vi "Write Single Coil1.vi"(7 "Unit_ID":T1, 8 "error in (no error)":errorcluster, 9 "coil value":bool, 10 "address":u16, 11 "Modbus master in":refnum<class "TCP.lvclass">) -> (0 "error out":errorcluster, 3 "Modbus master out":refnum<class "TCP.lvclass">)   [LabVIEW 2019, in "NI_modbus_upd.lvlib"]
doc: "Writes a value to a single coil."
uses:
  NI_modbus_upd.lvlib
  TCP/TCP.lvclass
  Ctl/Unit_ID.ctl
  TCP/TCP.lvclass/TCP.ctl
  Error Generator1.vi
  Function code mismatch error1.vi
  Read ADU Packet Master.vi
  Write ADU Packet Master.vi
  Modbus Data Unit (PDU)/Construct PDU1.vi
  Modbus Data Unit (PDU)/Unflatten to PDU1.vi
  TCP/Protocol Read.vi
  TCP/Protocol Write.vi
  <vilib>/Utility/error.llb/Error Cluster From Error Code.vi
  Modbus Data Unit (PDU)/Deconstruct PDU1.vi
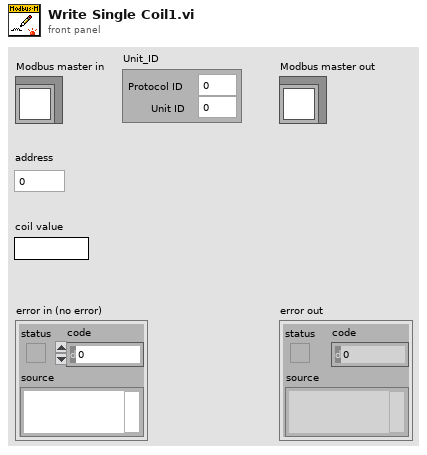
[diagram p1: front panel]
types:
  T1 = typedef "NI_modbus_upd.lvlib/Unit_ID.ctl" = cluster{"Protocol ID":u16, "Unit ID":u8}
  T2 = typedef "NI_modbus_upd.lvlib/MB Modbus Data Unit.ctl" = cluster{"function":T3, "Data":u8[]}
  T3 = typedef "NI_modbus_upd.lvlib/Function.ctl" = u8
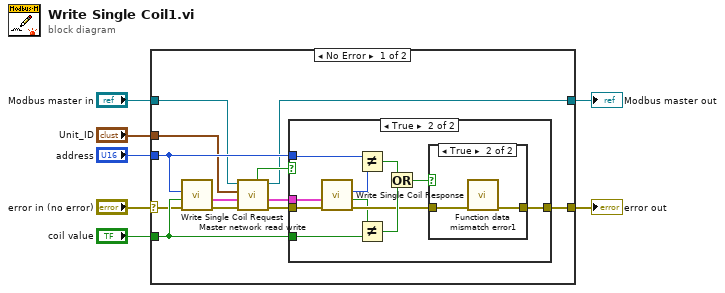
[diagram p0: block diagram]
diagram:
  n1 = case shown="No Error" "error in (no error)" {
    selector: "error in (no error)" -> [w9 w36]
    tunnel: "Modbus master in" -> [w12 w35]
    tunnel: [w18 w36] -> w4
    tunnel: [w13 w35] -> w3
    tunnel: "address" -> [w15 _]
    tunnel: "coil value" -> [w17 _]
    tunnel: "Unit_ID" -> [w10 _]
    frame No Error {
      n2 = call "Write Single Coil Request.vi"("error in (no error)"=w9, "coil value"=w17, "starting address"=w15) -> ("error out"=w19:errorcluster, "Modbus Data Unit out"=w11:T2)  [unwired: 7 in]
      n3 = call "Master network read write.vi"("error in (no error)"=w19, "Modbus Data Unit"=w11, "Unit_ID"=w10, "TCP in"=w12) -> ("error out"=w16:errorcluster, "Modbus data unit out"=w8:T2, "TCP out"=w13:refnum<class "TCP.lvclass">, "PDU valid?"=w14:bool)  [unwired: 4 in]
      n4 = case shown="True" w14 {
        tunnel: [w20 w30] -> w18
        tunnel: w17 -> [_ w23]
        tunnel: w16 -> [w20 w26]
        tunnel: w15 -> [_ w24]
        tunnel: w8 -> [_ w21]
        frame False {
        }
        frame True {
          n5 = call "Write Single Coil Response.vi"("error in (no error)"=w26, "Modbus Data Unit in"=w21) -> ("error out"=w25:errorcluster, "coil value"=w22:bool, "address"=w27:u16)  [unwired: 7 in]
          n6 = Not Equal?(x=w24, y=w27) -> (x != y?=w29:bool)
          n7 = Not Equal?(x=w22, y=w23) -> (x != y?=w28:bool)
          n8 = Or(x=w29, y=w28) -> (x .or. y?=w31:bool)
          n9 = case shown="True" w31 {
            tunnel: [w32 w34] -> w30
            tunnel: w25 -> [w32 w33]
            frame False {
            }
            frame True {
              n10 = call "Function data mismatch error1.vi"("error in (no error)"=w33) -> ("error out"=w34:errorcluster)  [unwired: 10 in]
            }
          }
        }
      }
    }
    frame Error {
    }
  }
  "error out" <- w4
  "Modbus master out" <- w3
